vi "SetPoint.vi"(8 "error in (no error)":errorcluster, 10 "Point":refnum<class "Point.lvclass">, 11 "Line in":refnum<class "Line.lvclass">) -> (0 "error out":errorcluster, 3 "Line out":refnum<class "Line.lvclass">)   [LabVIEW 2021, in "Picture2D.lvlib" / "Line.lvclass"]
uses:
  Line.lvclass
  Shape/Shape.lvclass
  Point/Point.lvclass
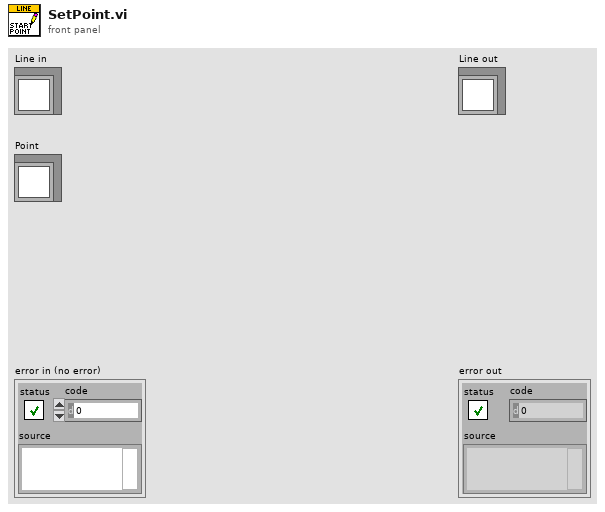
[diagram p1: front panel]
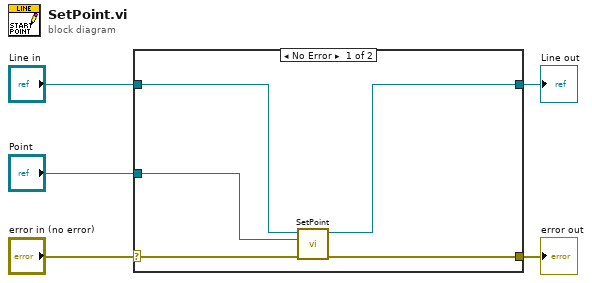
[diagram p0: block diagram]
diagram:
  n1 = case shown="No Error" "error in (no error)" {
    selector: "error in (no error)" -> [w10 w11]
    tunnel: [w9 w11] -> w4
    tunnel: [w6 w12] -> w2
    tunnel: "Line in" -> [w8 w12]
    tunnel: "Point" -> [w7 _]
    frame No Error {
      n2 = call-parent "SetPoint.vi"("error in (no error)"=w10, "Point"=w7, "Picture2D in"=w8) -> ("error out"=w9:errorcluster, "Picture2D out"=w6:refnum<class "Line.lvclass">)  [unwired: 7 in]
    }
    frame Error {
    }
  }
  "error out" <- w4
  "Line out" <- w2
